vi "Project.vi"() -> ()   [LabVIEW 2016]
uses:
  <vilib>/DAQmx/read.llb/DAQmx Read (Digital Bool 1Line 1Point).vi
  <vilib>/DAQmx/write.llb/DAQmx Write (Digital Bool 1Line 1Point).vi
  <vilib>/DAQmx/create/channels.llb/DAQmx Create Channel (DI-Digital Input).vi
  <vilib>/DAQmx/create/channels.llb/DAQmx Create Channel (DO-Digital Output).vi
  <vilib>/DAQmx/miscellaneous.llb/DAQmx Fill In Error Info.vi
panel:
  in  "stop":bool
  out "Conveyor":bool
  out "STOP":bool
  out "START":bool
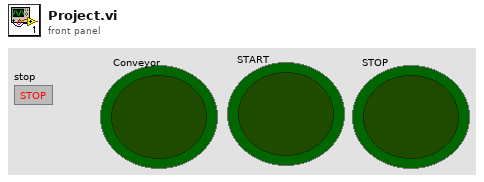
[diagram p1: front panel]
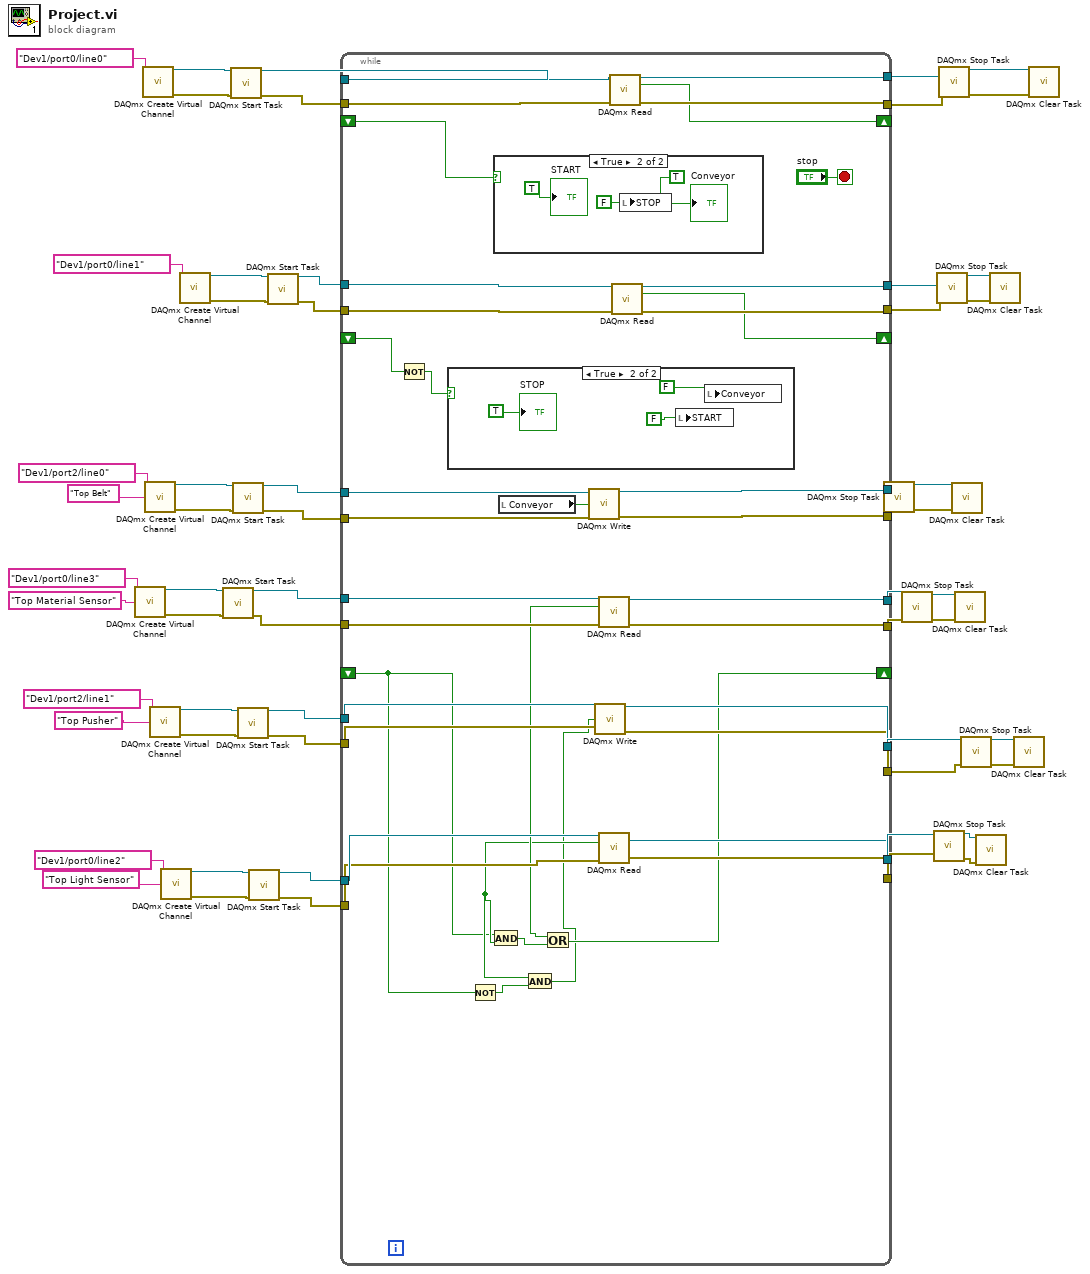
[diagram p0: block diagram]
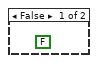
[diagram p2: hidden frame]
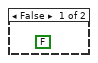
[diagram p3: hidden frame]
diagram:
  n1 = call-poly <vilib>:"DAQmx Create Virtual Channel.vi"("lines"=tag "Dev1/port0/line3", "name to assign"="Top Material Sensor") -> ("task out"=w31:refnum<k21>, "error out"=w30:errorcluster)  [unwired: 12 in]
  n2 = call-poly <vilib>:"DAQmx Create Virtual Channel.vi"("lines"=tag "Dev1/port0/line0") -> ("task out"=w58:refnum<k21>, "error out"=w57:errorcluster)  [unwired: 13 in]
  n3 = call-poly <vilib>:"DAQmx Create Virtual Channel.vi"("lines"=tag "Dev1/port2/line0", "name to assign"="Top Belt") -> ("task out"=w42:refnum<k21>, "error out"=w41:errorcluster)  [unwired: 12 in]
  n4 = call-poly <vilib>:"DAQmx Create Virtual Channel.vi"("lines"=tag "Dev1/port2/line1", "name to assign"="Top Pusher") -> ("task out"=w18:refnum<k21>, "error out"=w17:errorcluster)  [unwired: 12 in]
  n5 = call-poly <vilib>:"DAQmx Create Virtual Channel.vi"("lines"=tag "Dev1/port0/line2", "name to assign"="Top Light Sensor") -> ("task out"=w9:refnum<k21>, "error out"=w8:errorcluster)  [unwired: 12 in]
  n6 = call-poly <vilib>:"DAQmx Create Virtual Channel.vi"("lines"=tag "Dev1/port0/line1") -> ("task out"=w50:refnum<k21>, "error out"=w49:errorcluster)  [unwired: 13 in]
  n7 = call <vilib>:"DAQmx Start Task.vi"("task/channels in"=w31, "error in"=w30) -> ("task out"=w28:refnum<k21>, "error out"=w27:errorcluster)  [unwired: 12 in]
  n8 = call <vilib>:"DAQmx Start Task.vi"("task/channels in"=w58, "error in"=w57) -> ("task out"=w56:refnum<k21>, "error out"=w55:errorcluster)  [unwired: 12 in]
  n9 = call <vilib>:"DAQmx Start Task.vi"("task/channels in"=w42, "error in"=w41) -> ("task out"=w40:refnum<k21>, "error out"=w39:errorcluster)  [unwired: 12 in]
  n10 = call <vilib>:"DAQmx Start Task.vi"("task/channels in"=w18, "error in"=w17) -> ("task out"=w15:refnum<k21>, "error out"=w14:errorcluster)  [unwired: 12 in]
  n11 = call <vilib>:"DAQmx Start Task.vi"("task/channels in"=w9, "error in"=w8) -> ("task out"=w6:refnum<k21>, "error out"=w5:errorcluster)  [unwired: 12 in]
  n12 = call <vilib>:"DAQmx Start Task.vi"("task/channels in"=w50, "error in"=w49) -> ("task out"=w46:refnum<k21>, "error out"=w45:errorcluster)  [unwired: 12 in]
  n13 = while {
    tunnel: w56 -> [w96]
    tunnel: w55 -> [w95]
    tunnel: [w94] -> w54
    tunnel: [w93] -> w53
    shift-right: [w92] -> _
    shift-left: _ -> [w91]
    tunnel: w46 -> [w90]
    tunnel: w45 -> [w89]
    tunnel: [w88] -> w44
    tunnel: [w87] -> w43
    shift-right: [w86] -> _
    shift-left: _ -> [w85]
    tunnel: w40 -> [w83]
    tunnel: w39 -> [w82]
    tunnel: [w81] -> w36
    tunnel: [w80] -> w35
    tunnel: w28 -> [w77]
    tunnel: w27 -> [w76]
    tunnel: [w75] -> w24
    tunnel: [w74] -> w23
    tunnel: [w71] -> w20
    tunnel: [w70] -> w19
    tunnel: w15 -> [w73]
    tunnel: w14 -> [w72]
    tunnel: [w66] -> w11
    tunnel: [w67] -> w10
    tunnel: w6 -> [w69]
    tunnel: w5 -> [w68]
    shift-right: [w65] -> _
    shift-left: _ -> [w61]
    stop <- "stop" stop-if-true
    n14 = Not(x=w85) -> (.not. x?=w84:bool)
    n15 = case shown="True" w84 {
      frame False {
        (unwired) FALSE
      }
      frame True {
        n16 = local write "START"(FALSE) -> ()
        n17 = local write "Conveyor"(FALSE) -> ()
        "STOP" <- TRUE
      }
    }
    n18 = Not(x=w61) -> (.not. x?=w60:bool)
    n19 = case shown="True" w91 {
      frame False {
        (unwired) FALSE
      }
      frame True {
        n20 = local write "STOP"(FALSE) -> ()
        "START" <- TRUE
        "Conveyor" <- TRUE
      }
    }
    n21 = local read "Conveyor"() -> (w78:bool)
    n22 = call-poly <vilib>:"DAQmx Write.vi"("task/channels in"=w83, "data"=w78, "error in"=w82) -> ("task out"=w81:refnum<k21>, "error out"=w80:errorcluster)  [unwired: 10 in, 1 out]
    n23 = call-poly <vilib>:"DAQmx Read.vi"("task/channels in"=w77, "error in"=w76) -> ("task out"=w75:refnum<k21>, "data"=w64:bool, "error out"=w74:errorcluster)  [unwired: 11 in]
    n24 = call-poly <vilib>:"DAQmx Read.vi"("task/channels in"=w69, "error in"=w68) -> ("task out"=w66:refnum<k21>, "data"=w62:bool, "error out"=w67:errorcluster)  [unwired: 11 in]
    n25 = And(x=w61, y=w62) -> (x .and. y?=w63:bool)
    n26 = And(x=w62, y=w60) -> (x .and. y?=w59:bool)
    n27 = Or(x=w64, y=w63) -> (x .or. y?=w65:bool)
    n28 = call-poly <vilib>:"DAQmx Write.vi"("task/channels in"=w73, "data"=w59, "error in"=w72) -> ("task out"=w71:refnum<k21>, "error out"=w70:errorcluster)  [unwired: 10 in, 1 out]
    n29 = call-poly <vilib>:"DAQmx Read.vi"("task/channels in"=w96, "error in"=w95) -> ("task out"=w94:refnum<k21>, "data"=w92:bool, "error out"=w93:errorcluster)  [unwired: 11 in]
    n30 = call-poly <vilib>:"DAQmx Read.vi"("task/channels in"=w90, "error in"=w89) -> ("task out"=w87:refnum<k21>, "data"=w86:bool, "error out"=w88:errorcluster)  [unwired: 11 in]
  }
  n31 = call <vilib>:"DAQmx Stop Task.vi"("task/channels in"=w36, "error in"=w35) -> ("task out"=w38:refnum<k21>, "error out"=w37:errorcluster)  [unwired: 12 in]
  n32 = call <vilib>:"DAQmx Stop Task.vi"("task/channels in"=w24, "error in"=w23) -> ("task out"=w26:refnum<k21>, "error out"=w25:errorcluster)  [unwired: 12 in]
  n33 = call <vilib>:"DAQmx Stop Task.vi"("task/channels in"=w11, "error in"=w10) -> ("task out"=w13:refnum<k21>, "error out"=w12:errorcluster)  [unwired: 12 in]
  n34 = call <vilib>:"DAQmx Stop Task.vi"("task/channels in"=w43, "error in"=w44) -> ("task out"=w48:refnum<k21>, "error out"=w47:errorcluster)  [unwired: 12 in]
  n35 = call <vilib>:"DAQmx Stop Task.vi"("task/channels in"=w54, "error in"=w53) -> ("task out"=w52:refnum<k21>, "error out"=w51:errorcluster)  [unwired: 12 in]
  n36 = call <vilib>:"DAQmx Clear Task.vi"("task in"=w38, "error in"=w37) -> ()  [unwired: 13 in, 1 out]
  n37 = call <vilib>:"DAQmx Clear Task.vi"("task in"=w26, "error in"=w25) -> ()  [unwired: 13 in, 1 out]
  n38 = call <vilib>:"DAQmx Stop Task.vi"("task/channels in"=w20, "error in"=w19) -> ("task out"=w22:refnum<k21>, "error out"=w21:errorcluster)  [unwired: 12 in]
  n39 = call <vilib>:"DAQmx Clear Task.vi"("task in"=w13, "error in"=w12) -> ()  [unwired: 13 in, 1 out]
  n40 = call <vilib>:"DAQmx Clear Task.vi"("task in"=w48, "error in"=w47) -> ()  [unwired: 13 in, 1 out]
  n41 = call <vilib>:"DAQmx Clear Task.vi"("task in"=w22, "error in"=w21) -> ()  [unwired: 13 in, 1 out]
  n42 = call <vilib>:"DAQmx Clear Task.vi"("task in"=w52, "error in"=w51) -> ()  [unwired: 13 in, 1 out]
